vi "DrawTextOnWavefomrAndXYPlots.vi"(0 "xy plot In":picture, 1 "Text To Draw":string, 2 "desired font(Application)":T1(ring), 3 "[user-specified font]":T2={"Font Name:"="Current Font", "Size"=36, "Strikeout?"=FALSE, "Italic?"=FALSE, "Underline?"=FALSE, "Outline?"=TRUE, "Shadow?"=TRUE, "Bold?"=TRUE}, 4 "waveform plot In":picture) -> (5 "waveform plot Out":picture, 6 "xy plot Out":picture)   [LabVIEW 2012]
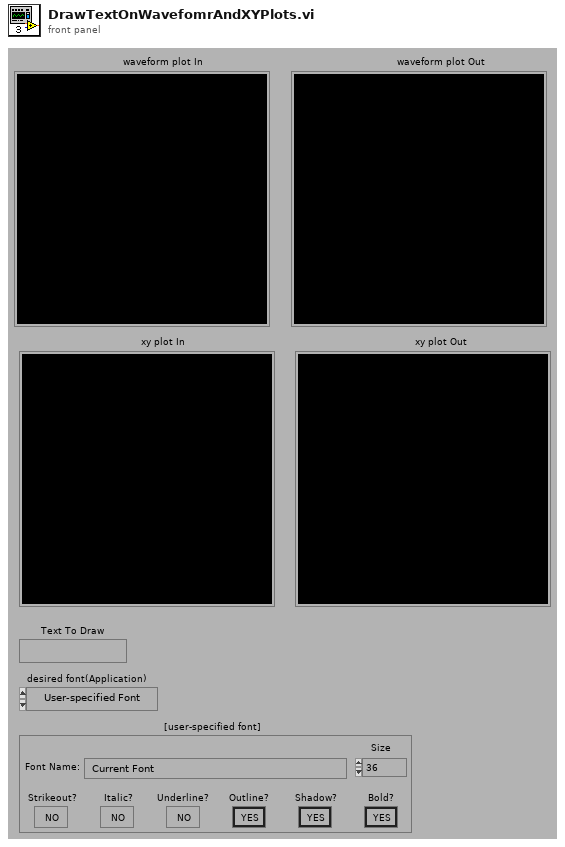
[diagram p1: front panel]
types:
  T1 = enum16{"User-specified Font", "Application Font", "System Font", "Dialog Font"}
  T2 = cluster{"Font Name:":string, "Size":i16, "Strikeout?":bool, "Italic?":bool, "Underline?":bool, "Outline?":bool, "Shadow?":bool, "Bold?":bool}
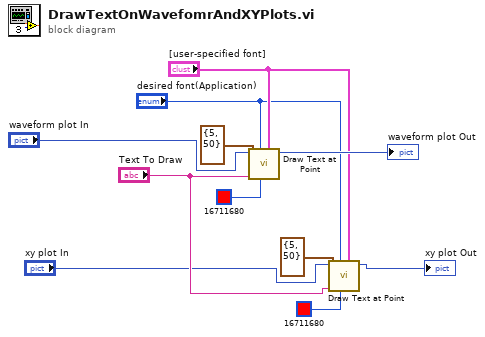
[diagram p0: block diagram]
diagram:
  n1 = call <vilib>:"Draw Text at Point.vi"("[user-specified font]"="[user-specified font]", "text color(black)"=u32 16711680, "desired font(Application)"="desired font(Application)", "text"="Text To Draw", "origin"=cluster{"x":i16, "y":i16} {"x"=5, "y"=50}, "picture"="waveform plot In") -> ("new picture"=→"waveform plot Out":picture)  [unwired: 3 in, 2 out]
  n2 = call <vilib>:"Draw Text at Point.vi"("[user-specified font]"="[user-specified font]", "text color(black)"=u32 16711680, "desired font(Application)"="desired font(Application)", "text"="Text To Draw", "origin"=cluster{"x":i16, "y":i16} {"x"=5, "y"=50}, "picture"="xy plot In") -> ("new picture"=→"xy plot Out":picture)  [unwired: 3 in, 2 out]
